vi "Add Sections.vi"(8 "error in":errorcluster, 10 "Section in":refnum<class "Section.lvclass">[](array[class]), 11 "Node Ptr in":T1 format="%.0x") -> (0 "error out":errorcluster, 3 "Node Ptr out":T1 format="%.0x")   [LabVIEW 2024, in "FPGA Addon System Explorer.lvlib"]
uses:
  FPGA Addon System Explorer.lvlib
  <vilib>/NI VeriStand/Custom Device API/Custom Device Item Ref.ctl
  Parser/Section/Section.lvclass
  <vilib>/NI VeriStand/Custom Device API/Custom Device API.lvlib
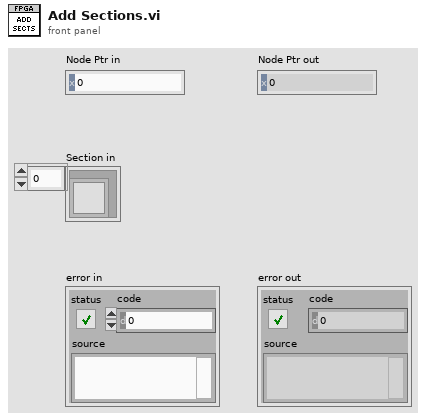
[diagram p1: front panel]
types:
  T1 = typedef "Custom Device API.lvlib/Custom Device Item Ref.ctl" = u64
  T2 = cluster{"Name":string, "TypeGUID":string, "Identifier":string}
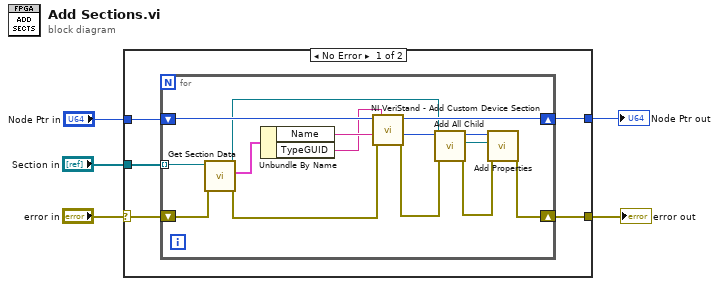
[diagram p0: block diagram]
diagram:
  n1 = case shown="No Error" "error in" {
    selector: "error in" -> [w9 w27]
    tunnel: [w10 w27] -> w5
    tunnel: "Node Ptr in" -> [w8 w26]
    tunnel: [w7 w26] -> w2
    tunnel: "Section in" -> [w6 _]
    frame No Error {
      n2 = for {
        tunnel: w6 -> [w19] mode=indexing
        shift-right: [w23] -> w10
        shift-left: w9 -> [w25]
        shift-right: [w17] -> w7
        shift-left: w8 -> [w18]
        n3 = call "Get Section Data.vi"("error in"=w25, "Section in"=w19) -> ("error out"=w24:errorcluster, "Section Data"=w20:T2, "Section out"=w12:refnum<class "Section.lvclass">)  [unwired: 7 in]
        n4 = Unbundle By Name(w20) -> ("Name"=w13:string, "TypeGUID"=w11:string)
        n5 = call <vilib>:"NI VeriStand - Add Custom Device Section.vi"("GUID (Default Section)"=w11, "error in (no error)"=w24, "Section Name"=w13, "Parent Ref in"=w18) -> ("error out"=w22:errorcluster, "Section Ptr"=w15:T1, "Parent Ref out"=w17:T1)  [unwired: 4 in, 1 out]
        n6 = call "Add All Child.vi"("error in"=w22, "Item in"=w12, "Parent Ref in"=w15) -> ("error out"=w21:errorcluster, "Item out"=w16:refnum<class "Section.lvclass">, "Parent Ref out"=w14:T1)  [unwired: 6 in]
        n7 = call "Add Properties.vi"("error in"=w21, "Item in"=w16, "Node Ptr in"=w14) -> ("error out"=w23:errorcluster)  [unwired: 7 in, 1 out]
      }
    }
    frame Error {
    }
  }
  "error out" <- w5
  "Node Ptr out" <- w2
